vi "Enum Server.vi"() -> ()   [LabVIEW 2020]
uses:
  source/PV Data/NT Enum/NT Enum.lvclass
  source/Server/Server/Server.lvclass
  source/PV Data/PV Data.lvlib
  source/Server/Server/Fetch (NT Enum).vi
  source/Server/Server/Post (NT Enum (Index & Choices)).vi
  source/Server/Server/Add PV (NT Enum (Index & Choices)).vi
  source/PV Data/NT Enum/Configure Control (Ring).vi
  source/Server/Server/Add PV (NT Enum (Reference)).vi
  source/Server/Server/Add PV (NT Enum (Enum)).vi
  source/Server/Server/Post (NT).vi
panel:
  in  "Enum":enum16{"A", "B", "C"}(ring)
  in  "Ring":u16(ring) items=["A", "B", "C"]
  in  "index":u16=1
  in  "choices":string[](array[string])=["A", "B", "C"]
  in  "stop":bool
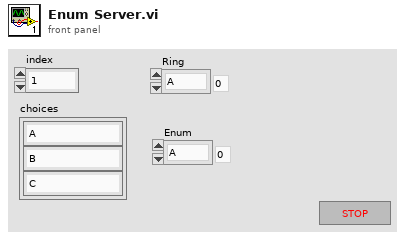
[diagram p1: front panel]
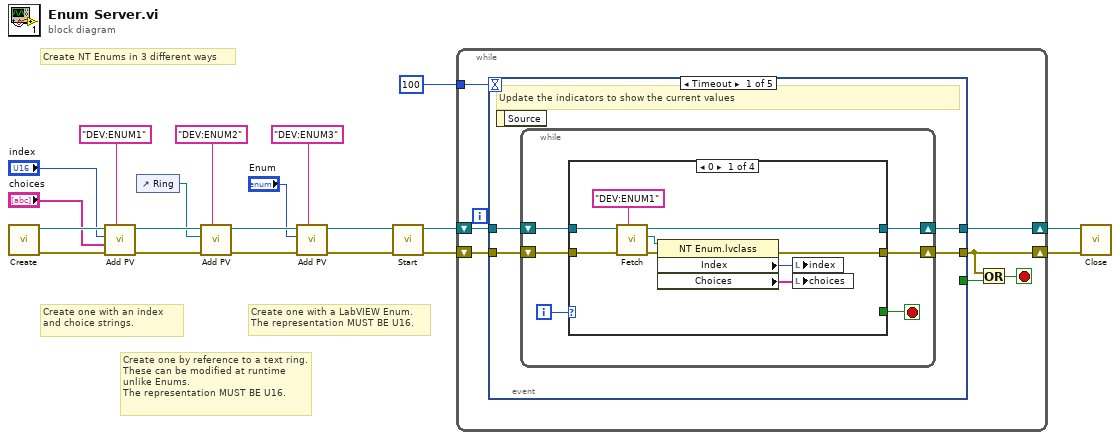
[diagram p0: block diagram]
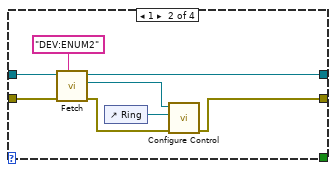
[diagram p2: hidden frame]
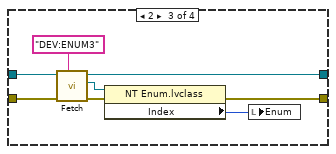
[diagram p3: hidden frame]
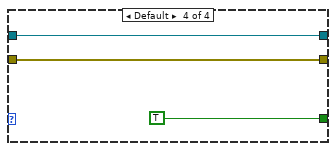
[diagram p4: hidden frame]
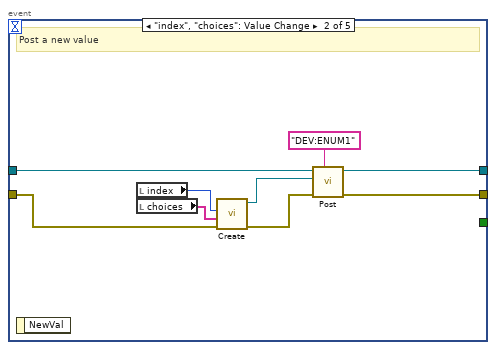
[diagram p5: hidden frame]
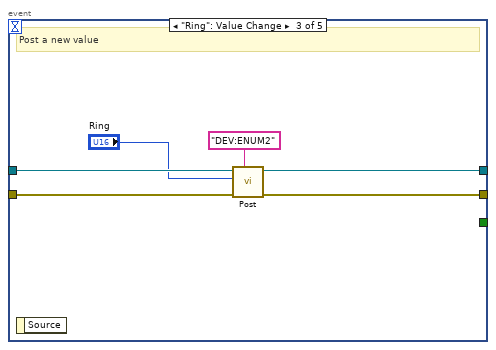
[diagram p6: hidden frame]
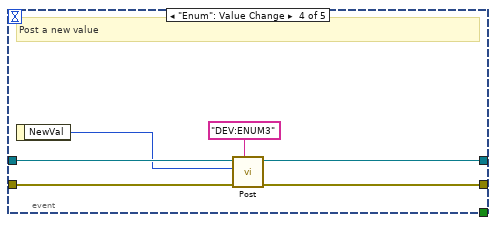
[diagram p7: hidden frame]
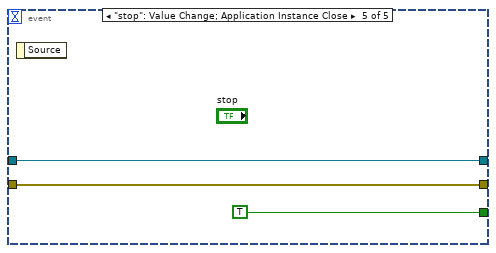
[diagram p8: hidden frame]
diagram:
  # "Create one with a LabVIEW Enum.\nThe representation MUST BE U16."
  # "Create one by reference to a text ring. These can be modified at runtime unlike Enums.\nThe representation MUST BE U16."
  # "Create one with an index and choice strings."
  # "Create NT Enums in 3 different ways"
  n1 = call "Create.vi"() -> ("error out"=w14:errorcluster, "Server out"=w17:refnum<class "Server.lvclass">)  [unwired: 10 in]
  n2 = call-poly "Add PV.vi"("PV name"="DEV:ENUM1", "error in (no error)"=w14, "initial choices"="choices", "initial index"="index", "Server in"=w17) -> ("error out"=w6:errorcluster, "Server out"=w11:refnum<class "Server.lvclass">)  [unwired: 2 in, 3 out]
  n3 = control-ref of="Ring"() -> (w5:refnum<vi>)
  n4 = call-poly "Add PV.vi"("PV name"="DEV:ENUM2", "error in (no error)"=w6, "ref"=w5, "Server in"=w11) -> ("error out"=w7:errorcluster, "Server out"=w10:refnum<class "Server.lvclass">)  [unwired: 4 in, 2 out]
  n5 = call-poly "Add PV.vi"("PV name"="DEV:ENUM3", "error in (no error)"=w7, "initial value"="Enum", "Server in"=w10) -> ("error out"=w8:errorcluster, "Server out"=w9:refnum<class "Server.lvclass">)  [unwired: 4 in, 2 out]
  n6 = call-dynamic "Start.vi"("error in (no error)"=w8, "Server in"=w9) -> ("error out"=w1:errorcluster, "Server out"=w15:refnum<class "Server.lvclass">)  [unwired: 8 in]
  n7 = while {
    shift-right: [w25] -> w18
    shift-left: w15 -> [w26]
    shift-right: [w22] -> w19
    shift-left: w1 -> [w27]
    tunnel: 100 ("Numeric") -> [w21]
    stop <- w23 stop-if-true
    n8 = event shown="[0] Timeout" {
      selector: _ -> [_ _ _ _ _]
      dyn-events: _ -> [_ _ _ _ _]
      timeout: w21 -> [_ _ _ _ _]
      tunnel: w27 -> [w31 w71 w76 w82 w88]
      tunnel: w26 -> [w30 w74 w80 w86 w87]
      tunnel: [w28 w72 w78 w84 w88] -> w22
      tunnel: [w29 w73 w79 w85 w87] -> w25
      tunnel: [_ _ _ _ TRUE] -> w24
      event Timeout {
        # "Update the indicators to show the current values"
        n9 = event-data() -> ()  [unwired: 1 in, 1 out]
        n10 = while {
          shift-right: [w34] -> w28
          shift-left: w31 -> [w37]
          shift-right: [w35] -> w29
          shift-left: w30 -> [w36]
          i -> [w33]
          stop <- w32 stop-if-true
          n11 = case shown="0" w33 {
            tunnel: w37 -> [w46 w54 w62 w65]
            tunnel: w36 -> [w45 w53 w61 w64]
            tunnel: [w43 w49 w60 w64] -> w35
            tunnel: [w40 w51 w56 w65] -> w34
            tunnel: [_ _ _ TRUE] -> w32
            frame 0 {
              n12 = call-poly "Fetch.vi"("PV name"="DEV:ENUM1", "error in"=w46, "Server in"=w45) -> ("error out"=w44:errorcluster, "value"=w42:refnum<class "NT Enum.lvclass">, "Server out"=w43:refnum<class "Server.lvclass">)  [unwired: 6 in]
              n13 = property class="NT Enum.lvclass"(reference=w42, error in=w44) -> (error out=w40:errorcluster, "Index"=w41:u16, "Choices"=w39:string[])  [unwired: 1 out]
              n14 = local write "index"(w41) -> ()
              n15 = local write "choices"(w39) -> ()
            }
            frame 1 {
              n16 = call-poly "Fetch.vi"("PV name"="DEV:ENUM2", "error in"=w54, "Server in"=w53) -> ("error out"=w52:errorcluster, "value"=w50:refnum<class "NT Enum.lvclass">, "Server out"=w49:refnum<class "Server.lvclass">)  [unwired: 6 in]
              n17 = control-ref of="Ring"() -> (w47:refnum<vi>)
              n18 = call-poly "Configure Control.vi"("error in (no error)"=w52, "control"=w47, "NT Enum in"=w50) -> ("error out"=w51:errorcluster)  [unwired: 6 in, 2 out]
            }
            frame 2 {
              n19 = call-poly "Fetch.vi"("PV name"="DEV:ENUM3", "error in"=w62, "Server in"=w61) -> ("error out"=w58:errorcluster, "value"=w57:refnum<class "NT Enum.lvclass">, "Server out"=w60:refnum<class "Server.lvclass">)  [unwired: 6 in]
              n20 = property class="NT Enum.lvclass"(reference=w57, error in=w58) -> (error out=w56:errorcluster, "Index"=w55:u16)  [unwired: 1 out]
              n21 = local write "Enum"(w55) -> ()
            }
            frame Default {
            }
          }
        }
      }
      event "index", "choices": Value Change {
        # "Post a new value"
        n22 = event-data() -> ()  [unwired: 1 in, 1 out]
        n23 = local read "index"() -> (w67:u16)
        n24 = local read "choices"() -> (w68:string[])
        n25 = call-poly "Create.vi"("error in (no error)"=w71, "choices"=w68, "initial index"=w67) -> ("error out"=w70:errorcluster, "NT Enum out"=w69:refnum<class "NT Enum.lvclass">)  [unwired: 4 in, 3 out]
        n26 = call-poly "Post.vi"("PV name"="DEV:ENUM1", "error in (no error)"=w70, "value in"=w69, "Server in"=w74) -> ("error out"=w72:errorcluster, "Server out"=w73:refnum<class "Server.lvclass">)  [unwired: 5 in, 1 out]
      }
      event "Ring": Value Change {
        # "Post a new value"
        n27 = event-data() -> ()  [unwired: 1 in, 1 out]
        n28 = call-poly "Post.vi"("PV name"="DEV:ENUM2", "error in (no error)"=w76, "value in"="Ring", "Server in"=w80) -> ("error out"=w78:errorcluster, "Server out"=w79:refnum<class "Server.lvclass">)  [unwired: 3 in, 3 out]
      }
      event "Enum": Value Change {
        # "Post a new value"
        n29 = event-data() -> ("NewVal"=w81:enum16{"A", "B", "C"})  [unwired: 1 in]
        n30 = call-poly "Post.vi"("PV name"="DEV:ENUM3", "error in (no error)"=w82, "value in"=w81, "Server in"=w86) -> ("error out"=w84:errorcluster, "Server out"=w85:refnum<class "Server.lvclass">)  [unwired: 3 in, 3 out]
      }
      event "stop": Value Change; Application Instance Close {
        n31 = event-data() -> ()  [unwired: 1 in, 1 out]
      }
    }
    n32 = Or(x=w22, y=w24) -> (x .or. y?=w23:bool)
  }
  n33 = call-dynamic "Close.vi"("error in"=w19, "Server in"=w18) -> ()  [unwired: 9 in, 1 out]
